vi "Test Asic Rate Scan Adders.vi"(8 "Error IN":errorcluster, 11 "Config Test IN":T2={"Config HW"={"VISA Rigol DP832"="Rigol_DP832", "Config Rigol DP832"=[{"Channel"=0, "V Limit"=5.5, "I Limit"=0.5, "V Out"=5.0}, {"Channel"=1, "V Limit"=5.5, "I Limit"=0.8, "V Out"=5.0}, {"Channel"=2, "V Limit"=5.5, "I Limit"=0.2, "V Out"=0.0}], "CTA Test#"="CTA013 A", "FT_Handle"=0, "Espera acceso FT"=10, "VISA Tek MDO3104"="Rigol_DP832", "VISA Key 81160A"="Rigol_DP832"}, "Config Test"=[{"Vasic"=2.8, "Global Reset"=FALSE, "Test Register?"=FALSE, "Test ADC?"=FALSE, "Test ADC"={"Repeats ADC"=100, "Max Desviation"=0.1}, "Limits ADC"={"Low"=[1.9, 1.3, 0.65, 0.0, 1.6, 1.4, 1.4, 0.9, 2.1, 0.85, 1.9], "High"=[2.1, 1.5, 0.85, 0.1, 1.4, 1.2, 1.2, 0.7, 1.9, 0.65, 1.7]}, "Test Max PN Min NP?"=FALSE, "Limits Max PN Min NP"={"Max P Upper"=2.177000045776367, "Min P Upper"=1.474, "Max N Upper"=1.475, "Min N Upper"=0.818, "Max P Lower"=1.888, "Min P Lower "=1.321, "Max N Lower"=1.322, "Min N Lower"=0.73}, "Test Rate Scan?"=FALSE, "Vin Rate Scan"=[], "Limits Rate Scan"={"High"=[0.15, 0.242, 0.331, 0.425, 0.512, 0.6, 0.688, 0.774, 0.847, 0.91], "Low"=[0.021, 0.11, 0.189, 0.27, 0.347, 0.421, 0.487, 0.551, 0.601, 0.635]}, "Test Rate Scan Adders?"=FALSE, "Vin Rate Adders"=[], "Limits Rate Scan adders"={"High"=[], "Low"=[]}, "Test offset analog?"=FALSE, "Lim Offset Analog"={"Max Analog"=0.05, "Min Analog"=-0.05}, "Test offset digital?"=FALSE, "Lim offset Dig"={"Max Dig"=0.05}, "Vasic real f.a."=2.8, "IBIAS"=FALSE, "VALUE IBIAS"=63}, {"Vasic"=2.8, "Global Reset"=FALSE, "Test Register?"=FALSE, "Test ADC?"=FALSE, "Test ADC"={"Repeats ADC"=100, "Max Desviation"=0.1}, "Limits ADC"={"Low"=[1.9, 1.3, 0.65, 0.0, 1.6, 1.4, 1.4, 0.9, 2.1, 0.85, 1.9], "High"=[2.1, 1.5, 0.85, 0.1, 1.4, 1.2, 1.2, 0.7, 1.9, 0.65, 1.7]}, "Test Max PN Min NP?"=FALSE, "Limits Max PN Min NP"={"Max P Upper"=2.177000045776367, "Min P Upper"=1.474, "Max N Upper"=1.475, "Min N Upper"=0.818, "Max P Lower"=1.888, "Min P Lower "=1.321, "Max N Lower"=1.322, "Min N Lower"=0.73}, "Test Rate Scan?"=FALSE, "Vin Rate Scan"=[], "Limits Rate Scan"={"High"=[0.15, 0.242, 0.331, 0.425, 0.512, 0.6, 0.688, 0.774, 0.847, 0.91], "Low"=[0.021, 0.11, 0.189, 0.27, 0.347, 0.421, 0.487, 0.551, 0.601, 0.635]}, "Test Rate Scan Adders?"=FALSE, "Vin Rate Adders"=[], "Limits Rate Scan adders"={"High"=[], "Low"=[]}, "Test offset analog?"=FALSE, "Lim Offset Analog"={"Max Analog"=0.05, "Min Analog"=-0.05}, "Test offset digital?"=FALSE, "Lim offset Dig"={"Max Dig"=0.05}, "Vasic real f.a."=2.8, "IBIAS"=FALSE, "VALUE IBIAS"=63}, {"Vasic"=2.8, "Global Reset"=FALSE, "Test Register?"=FALSE, "Test ADC?"=FALSE, "Test ADC"={"Repeats ADC"=100, "Max Desviation"=0.1}, "Limits ADC"={"Low"=[1.9, 1.3, 0.65, 0.0, 1.6, 1.4, 1.4, 0.9, 2.1, 0.85, 1.9], "High"=[2.1, 1.5, 0.85, 0.1, 1.4, 1.2, 1.2, 0.7, 1.9, 0.65, 1.7]}, "Test Max PN Min NP?"=FALSE, "Limits Max PN Min NP"={"Max P Upper"=2.177000045776367, "Min P Upper"=1.474, "Max N Upper"=1.475, "Min N Upper"=0.818, "Max P Lower"=1.888, "Min P Lower "=1.321, "Max N Lower"=1.322, "Min N Lower"=0.73}, "Test Rate Scan?"=FALSE, "Vin Rate Scan"=[], "Limits Rate Scan"={"High"=[0.15, 0.242, 0.331, 0.425, 0.512, 0.6, 0.688, 0.774, 0.847, 0.91], "Low"=[0.021, 0.11, 0.189, 0.27, 0.347, 0.421, 0.487, 0.551, 0.601, 0.635]}, "Test Rate Scan Adders?"=FALSE, "Vin Rate Adders"=[], "Limits Rate Scan adders"={"High"=[], "Low"=[]}, "Test offset analog?"=FALSE, "Lim Offset Analog"={"Max Analog"=0.05, "Min Analog"=-0.05}, "Test offset digital?"=FALSE, "Lim offset Dig"={"Max Dig"=0.05}, "Vasic real f.a."=2.8, "IBIAS"=FALSE, "VALUE IBIAS"=63}, {"Vasic"=2.8, "Global Reset"=FALSE, "Test Register?"=FALSE, "Test ADC?"=FALSE, "Test ADC"={"Repeats ADC"=100, "Max Desviation"=0.1}, "Limits ADC"={"Low"=[1.9, 1.3, 0.65, 0.0, 1.6, 1.4, 1.4, 0.9, 2.1, 0.85, 1.9], "High"=[2.1, 1.5, 0.85, 0.1, 1.4, 1.2, 1.2, 0.7, 1.9, 0.65, 1.7]}, "Test Max PN Min NP?"=FALSE, "Limits Max PN Min NP"={"Max P Upper"=2.177000045776367, "Min P Upper"=1.474, "Max N Upper"=1.475, "Min N Upper"=0.818, "Max P Lower"=1.888, "Min P Lower "=1.321, "Max N Lower"=1.322, "Min N Lower"=0.73}, "Test Rate Scan?"=FALSE, "Vin Rate Scan"=[], "Limits Rate Scan"={"High"=[0.15, 0.242, 0.331, 0.425, 0.512, 0.6, 0.688, 0.774, 0.847, 0.91], "Low"=[0.021, 0.11, 0.189, 0.27, 0.347, 0.421, 0.487, 0.551, 0.601, 0.635]}, "Test Rate Scan Adders?"=FALSE, "Vin Rate Adders"=[], "Limits Rate Scan adders"={"High"=[], "Low"=[]}, "Test offset analog?"=FALSE, "Lim Offset Analog"={"Max Analog"=0.05, "Min Analog"=-0.05}, "Test offset digital?"=FALSE, "Lim offset Dig"={"Max Dig"=0.05}, "Vasic real f.a."=2.8, "IBIAS"=FALSE, "VALUE IBIAS"=63}], "Result"=[], "Execucion Test"={"Vasic Actual"=0}, "Config VGA"={"Theoretical Voltage"=[], "Real Voltage"=[102.85, 207.14, 299.57, 404.85, 495.71, 606.85, 697.71, 801.14, 897.14, 998.85], "Pulse Width"=57344, "Frecuency Pulse"=1000000.0, "VGA Gain"=[9, 16, 24, 34, 43, 52, 61, 72, 81, 93]}, "Test Info"={"Asic"="", "Operator"="", "Place"="", "Time start"=timestamp(0 s since 1904-01-01), "Time stop"=timestamp(0 s since 1904-01-01)}, "Info machine"={"SO"="", "SO Name"="", "SO Ver"="", "SO Build"="", "CPU"="", "APP"="", "APP YEAR"="", "APP ver"="", "APP User"="", "APP Serail"="", "MAC"=[], "PC NAME"=[], "PC IP"=[], "BIOS MANU"="", "BIOS NAME"="", "BIOS SERIAL"="", "BOARD MANU"="", "BOARD NAME"="", "BOARD SERIAL"="", "Driver Version"="", "Library Version"="", "FPGA Ver"=0, "ID CTA board"=0, "LAST BOOT"="", "LABVIEW Ver"=0}, "Partial Report"="", "CONFIG GEN"=[]} {"CONFIG GEN"."Vasic Theorical" min=1.0 max=1000000.0 step=1.0 format="%#_6pV"; "CONFIG GEN"."Frequency" min=0.001 max=333000000.0 step=1000.0 format="%#_6pHz"; "CONFIG GEN"."Leading Edge Time" min=1e-09 max=1.0 step=1e-10 format="%#_6ps"; "CONFIG GEN"."Trailing Edge Time" min=1e-09 max=1.0 step=1e-10 format="%#_6ps"; "CONFIG GEN"."Delay" min=0.0 max=1.0 step=1e-12 format="%#_6ps"; "CONFIG GEN"."Trigger Level Sync" items=["ECL", "TTL"]; "CONFIG GEN"."Trigger Sync Out" items=["AB"=3, "B"=2, "A"=1, "None"=0]; "CONFIG GEN"."Load" min=1.0 max=1000000.0 step=1.0 format="%#_6p"; "CONFIG GEN"."DC Offset" min=-10.0 max=10.0 step=0.1 format="%#_6pV"; "CONFIG GEN"."Amplitude" min=0.05 max=5.0 step=0.001 format="%#_6pV"; "CONFIG GEN"."Width Time" min=1.5e-09 max=1.0 step=1e-10 format="%#_6ps"; "CONFIG GEN"."Channel" items=["Channel1"=1, "Channel2"=2]; "Config VGA"."Theoretical Voltage" format="%1.4f"; "Config VGA"."VGA Gain" format="%02x"; "Config VGA"."Frecuency Pulse" format="%0_2p"; "Config VGA"."Pulse Width" format="%04x"; "Config VGA"."Real Voltage" format="%1.5f"; "Config Test"."VALUE IBIAS" max=63 step=1; "Config Test"."Vasic real f.a." min=2.8 max=3.8 step=0.01 format="%.2g"; "Config Test"."Limits Rate Scan adders"."Low" format="%1.3f"; "Config Test"."Limits Rate Scan adders"."High" format="%1.3f"; "Config Test"."Limits ADC"."High" format="%1.4f"; "Config Test"."Limits ADC"."Low" format="%1.3f"; "Config Test"."Lim offset Dig"."Max Dig" format="%.3g"; "Config Test"."Lim Offset Analog"."Min Analog" format="%.3g"; "Config Test"."Lim Offset Analog"."Max Analog" format="%.3g"; "Config Test"."Limits Rate Scan"."Low" format="%1.4f"; "Config Test"."Limits Rate Scan"."High" format="%1.3f"; "Config Test"."Limits Max PN Min NP"."Min P Upper" format="%.3g"; "Config Test"."Limits Max PN Min NP"."Min P Lower" format="%.3g"; "Config Test"."Limits Max PN Min NP"."Max N Lower" format="%.3g"; "Config Test"."Limits Max PN Min NP"."Max N Upper" format="%.3g"; "Config Test"."Limits Max PN Min NP"."Min N Lower" format="%.3g"; "Config Test"."Limits Max PN Min NP"."Min N Upper" format="%.3g"; "Config Test"."Limits Max PN Min NP"."Max P Upper" format="%.3g"; "Config Test"."Limits Max PN Min NP"."Max P Lower" format="%.3g"; "Config Test"."Vasic" min=2.8 max=3.8 step=0.01 format="%.2g"; "Config HW"."Config Rigol DP832"."Channel" items=["+30V Channel 1", "+30V Channel 2", "+5V Channel 3"]; "Config HW"."Config Rigol DP832"."V Limit" format="%.1g"; "Config HW"."Config Rigol DP832"."I Limit" format="%.1g"; "Config HW"."Config Rigol DP832"."V Out" format="%.1g"; "Result"."Test Registros"."Read W/R" format="%04x"; "Result"."Test Registros"."Pattern W/R" format="%04x"; "Result"."Test Registros"."Read Default" format="%04x"; "Result"."Test Registros"."Pattern Default" format="%04x"}) -> (0 "Error OUT":errorcluster, 2 "Rate scan adders all ok":bool, 3 "Config Test OUT":T2={"Config HW"={"VISA Rigol DP832"="Rigol_DP832", "Config Rigol DP832"=[{"Channel"=0, "V Limit"=5.5, "I Limit"=0.5, "V Out"=5.0}, {"Channel"=1, "V Limit"=5.5, "I Limit"=0.8, "V Out"=5.0}, {"Channel"=2, "V Limit"=5.5, "I Limit"=0.2, "V Out"=0.0}], "CTA Test#"="CTA013 A", "FT_Handle"=0, "Espera acceso FT"=10, "VISA Tek MDO3104"="Rigol_DP832", "VISA Key 81160A"="Rigol_DP832"}, "Config Test"=[{"Vasic"=2.8, "Global Reset"=FALSE, "Test Register?"=FALSE, "Test ADC?"=FALSE, "Test ADC"={"Repeats ADC"=100, "Max Desviation"=0.1}, "Limits ADC"={"Low"=[1.9, 1.3, 0.65, 0.0, 1.6, 1.4, 1.4, 0.9, 2.1, 0.85, 1.9], "High"=[2.1, 1.5, 0.85, 0.1, 1.4, 1.2, 1.2, 0.7, 1.9, 0.65, 1.7]}, "Test Max PN Min NP?"=FALSE, "Limits Max PN Min NP"={"Max P Upper"=2.177000045776367, "Min P Upper"=1.474, "Max N Upper"=1.475, "Min N Upper"=0.818, "Max P Lower"=1.888, "Min P Lower "=1.321, "Max N Lower"=1.322, "Min N Lower"=0.73}, "Test Rate Scan?"=FALSE, "Vin Rate Scan"=[], "Limits Rate Scan"={"High"=[0.15, 0.242, 0.331, 0.425, 0.512, 0.6, 0.688, 0.774, 0.847, 0.91], "Low"=[0.021, 0.11, 0.189, 0.27, 0.347, 0.421, 0.487, 0.551, 0.601, 0.635]}, "Test Rate Scan Adders?"=FALSE, "Vin Rate Adders"=[], "Limits Rate Scan adders"={"High"=[], "Low"=[]}, "Test offset analog?"=FALSE, "Lim Offset Analog"={"Max Analog"=0.05, "Min Analog"=-0.05}, "Test offset digital?"=FALSE, "Lim offset Dig"={"Max Dig"=0.05}, "Vasic real f.a."=2.8, "IBIAS"=FALSE, "VALUE IBIAS"=63}, {"Vasic"=2.8, "Global Reset"=FALSE, "Test Register?"=FALSE, "Test ADC?"=FALSE, "Test ADC"={"Repeats ADC"=100, "Max Desviation"=0.1}, "Limits ADC"={"Low"=[1.9, 1.3, 0.65, 0.0, 1.6, 1.4, 1.4, 0.9, 2.1, 0.85, 1.9], "High"=[2.1, 1.5, 0.85, 0.1, 1.4, 1.2, 1.2, 0.7, 1.9, 0.65, 1.7]}, "Test Max PN Min NP?"=FALSE, "Limits Max PN Min NP"={"Max P Upper"=2.177000045776367, "Min P Upper"=1.474, "Max N Upper"=1.475, "Min N Upper"=0.818, "Max P Lower"=1.888, "Min P Lower "=1.321, "Max N Lower"=1.322, "Min N Lower"=0.73}, "Test Rate Scan?"=FALSE, "Vin Rate Scan"=[], "Limits Rate Scan"={"High"=[0.15, 0.242, 0.331, 0.425, 0.512, 0.6, 0.688, 0.774, 0.847, 0.91], "Low"=[0.021, 0.11, 0.189, 0.27, 0.347, 0.421, 0.487, 0.551, 0.601, 0.635]}, "Test Rate Scan Adders?"=FALSE, "Vin Rate Adders"=[], "Limits Rate Scan adders"={"High"=[], "Low"=[]}, "Test offset analog?"=FALSE, "Lim Offset Analog"={"Max Analog"=0.05, "Min Analog"=-0.05}, "Test offset digital?"=FALSE, "Lim offset Dig"={"Max Dig"=0.05}, "Vasic real f.a."=2.8, "IBIAS"=FALSE, "VALUE IBIAS"=63}, {"Vasic"=2.8, "Global Reset"=FALSE, "Test Register?"=FALSE, "Test ADC?"=FALSE, "Test ADC"={"Repeats ADC"=100, "Max Desviation"=0.1}, "Limits ADC"={"Low"=[1.9, 1.3, 0.65, 0.0, 1.6, 1.4, 1.4, 0.9, 2.1, 0.85, 1.9], "High"=[2.1, 1.5, 0.85, 0.1, 1.4, 1.2, 1.2, 0.7, 1.9, 0.65, 1.7]}, "Test Max PN Min NP?"=FALSE, "Limits Max PN Min NP"={"Max P Upper"=2.177000045776367, "Min P Upper"=1.474, "Max N Upper"=1.475, "Min N Upper"=0.818, "Max P Lower"=1.888, "Min P Lower "=1.321, "Max N Lower"=1.322, "Min N Lower"=0.73}, "Test Rate Scan?"=FALSE, "Vin Rate Scan"=[], "Limits Rate Scan"={"High"=[0.15, 0.242, 0.331, 0.425, 0.512, 0.6, 0.688, 0.774, 0.847, 0.91], "Low"=[0.021, 0.11, 0.189, 0.27, 0.347, 0.421, 0.487, 0.551, 0.601, 0.635]}, "Test Rate Scan Adders?"=FALSE, "Vin Rate Adders"=[], "Limits Rate Scan adders"={"High"=[], "Low"=[]}, "Test offset analog?"=FALSE, "Lim Offset Analog"={"Max Analog"=0.05, "Min Analog"=-0.05}, "Test offset digital?"=FALSE, "Lim offset Dig"={"Max Dig"=0.05}, "Vasic real f.a."=2.8, "IBIAS"=FALSE, "VALUE IBIAS"=63}, {"Vasic"=2.8, "Global Reset"=FALSE, "Test Register?"=FALSE, "Test ADC?"=FALSE, "Test ADC"={"Repeats ADC"=100, "Max Desviation"=0.1}, "Limits ADC"={"Low"=[1.9, 1.3, 0.65, 0.0, 1.6, 1.4, 1.4, 0.9, 2.1, 0.85, 1.9], "High"=[2.1, 1.5, 0.85, 0.1, 1.4, 1.2, 1.2, 0.7, 1.9, 0.65, 1.7]}, "Test Max PN Min NP?"=FALSE, "Limits Max PN Min NP"={"Max P Upper"=2.177000045776367, "Min P Upper"=1.474, "Max N Upper"=1.475, "Min N Upper"=0.818, "Max P Lower"=1.888, "Min P Lower "=1.321, "Max N Lower"=1.322, "Min N Lower"=0.73}, "Test Rate Scan?"=FALSE, "Vin Rate Scan"=[], "Limits Rate Scan"={"High"=[0.15, 0.242, 0.331, 0.425, 0.512, 0.6, 0.688, 0.774, 0.847, 0.91], "Low"=[0.021, 0.11, 0.189, 0.27, 0.347, 0.421, 0.487, 0.551, 0.601, 0.635]}, "Test Rate Scan Adders?"=FALSE, "Vin Rate Adders"=[], "Limits Rate Scan adders"={"High"=[], "Low"=[]}, "Test offset analog?"=FALSE, "Lim Offset Analog"={"Max Analog"=0.05, "Min Analog"=-0.05}, "Test offset digital?"=FALSE, "Lim offset Dig"={"Max Dig"=0.05}, "Vasic real f.a."=2.8, "IBIAS"=FALSE, "VALUE IBIAS"=63}], "Result"=[], "Execucion Test"={"Vasic Actual"=0}, "Config VGA"={"Theoretical Voltage"=[], "Real Voltage"=[102.85, 207.14, 299.57, 404.85, 495.71, 606.85, 697.71, 801.14, 897.14, 998.85], "Pulse Width"=57344, "Frecuency Pulse"=1000000.0, "VGA Gain"=[9, 16, 24, 34, 43, 52, 61, 72, 81, 93]}, "Test Info"={"Asic"="", "Operator"="", "Place"="", "Time start"=timestamp(0 s since 1904-01-01), "Time stop"=timestamp(0 s since 1904-01-01)}, "Info machine"={"SO"="", "SO Name"="", "SO Ver"="", "SO Build"="", "CPU"="", "APP"="", "APP YEAR"="", "APP ver"="", "APP User"="", "APP Serail"="", "MAC"=[], "PC NAME"=[], "PC IP"=[], "BIOS MANU"="", "BIOS NAME"="", "BIOS SERIAL"="", "BOARD MANU"="", "BOARD NAME"="", "BOARD SERIAL"="", "Driver Version"="", "Library Version"="", "FPGA Ver"=0, "ID CTA board"=0, "LAST BOOT"="", "LABVIEW Ver"=0}, "Partial Report"="", "CONFIG GEN"=[]} {"CONFIG GEN"."Vasic Theorical" min=1.0 max=1000000.0 step=1.0 format="%#_6pV"; "CONFIG GEN"."Frequency" min=0.001 max=333000000.0 step=1000.0 format="%#_6pHz"; "CONFIG GEN"."Leading Edge Time" min=1e-09 max=1.0 step=1e-10 format="%#_6ps"; "CONFIG GEN"."Trailing Edge Time" min=1e-09 max=1.0 step=1e-10 format="%#_6ps"; "CONFIG GEN"."Delay" min=0.0 max=1.0 step=1e-12 format="%#_6ps"; "CONFIG GEN"."Trigger Level Sync" items=["ECL", "TTL"]; "CONFIG GEN"."Trigger Sync Out" items=["AB"=3, "B"=2, "A"=1, "None"=0]; "CONFIG GEN"."Load" min=1.0 max=1000000.0 step=1.0 format="%#_6p"; "CONFIG GEN"."DC Offset" min=-10.0 max=10.0 step=0.1 format="%#_6pV"; "CONFIG GEN"."Amplitude" min=0.05 max=5.0 step=0.001 format="%#_6pV"; "CONFIG GEN"."Width Time" min=1.5e-09 max=1.0 step=1e-10 format="%#_6ps"; "CONFIG GEN"."Channel" items=["Channel1"=1, "Channel2"=2]; "Config VGA"."Theoretical Voltage" format="%1.4f"; "Config VGA"."VGA Gain" format="%02x"; "Config VGA"."Frecuency Pulse" format="%0_2p"; "Config VGA"."Pulse Width" format="%04x"; "Config VGA"."Real Voltage" format="%1.5f"; "Config Test"."VALUE IBIAS" max=63 step=1; "Config Test"."Vasic real f.a." min=2.8 max=3.8 step=0.01 format="%.2g"; "Config Test"."Limits Rate Scan adders"."Low" format="%1.3f"; "Config Test"."Limits Rate Scan adders"."High" format="%1.3f"; "Config Test"."Limits ADC"."High" format="%1.4f"; "Config Test"."Limits ADC"."Low" format="%1.3f"; "Config Test"."Lim offset Dig"."Max Dig" format="%.3g"; "Config Test"."Lim Offset Analog"."Min Analog" format="%.3g"; "Config Test"."Lim Offset Analog"."Max Analog" format="%.3g"; "Config Test"."Limits Rate Scan"."Low" format="%1.4f"; "Config Test"."Limits Rate Scan"."High" format="%1.3f"; "Config Test"."Limits Max PN Min NP"."Min P Upper" format="%.3g"; "Config Test"."Limits Max PN Min NP"."Min P Lower" format="%.3g"; "Config Test"."Limits Max PN Min NP"."Max N Lower" format="%.3g"; "Config Test"."Limits Max PN Min NP"."Max N Upper" format="%.3g"; "Config Test"."Limits Max PN Min NP"."Min N Lower" format="%.3g"; "Config Test"."Limits Max PN Min NP"."Min N Upper" format="%.3g"; "Config Test"."Limits Max PN Min NP"."Max P Upper" format="%.3g"; "Config Test"."Limits Max PN Min NP"."Max P Lower" format="%.3g"; "Config Test"."Vasic" min=2.8 max=3.8 step=0.01 format="%.2g"; "Config HW"."Config Rigol DP832"."Channel" items=["+30V Channel 1", "+30V Channel 2", "+5V Channel 3"]; "Config HW"."Config Rigol DP832"."V Limit" format="%.1g"; "Config HW"."Config Rigol DP832"."I Limit" format="%.1g"; "Config HW"."Config Rigol DP832"."V Out" format="%.1g"; "Result"."Test Registros"."Read W/R" format="%04x"; "Result"."Test Registros"."Pattern W/R" format="%04x"; "Result"."Test Registros"."Read Default" format="%04x"; "Result"."Test Registros"."Pattern Default" format="%04x"})   [LabVIEW 2019]
uses:
  Test.ctl
  TEST.TEST CONFIG HW.ctl
  Rigol DP832/DP832_Control Channels.ctl
  TEST.TEST CONFIG TEST MATRIZ.ctl
  TEST.TEST CONFIG TEST.ctl
  TEST.TEST RESULT.ctl
  test_result fvasic.ctl
  TEST.TEST EXECUTION TEST.ctl
  TEST.TEST CONFIG VGA.ctl
  TEST.TEST TEST INFO.ctl
  TEST.TEST INFO PC.ctl
  GenPulse_configurar.ctl
  Global.Salir Ya.vi
panel:
  out "Vin real gen":dbl[](array[numeric])
  in  "Debug":enum32{"Page 1", "Page 2"}(tab)
  in  "Operacion":enum32{"Page 1", "Page 2"}(tab)
  out "%":u8 format="%02d%%"
  out "B":u8(slide) scale=0.0..100.0
  out "Indicador":string
  out "HLTHx":dbl
  out "LLTHx":dbl
  out "WRITE OK":bool
  out "Amplitude":dbl
  in  "Column Headers":string[](array[string])=["MODE 2 (2+4)", "MODE 2 (3+4)", "MODE 2 (4+5)", "MODE 3 (2+3+4)", "MODE 3 (3+4+5)", "MODE 3 (4+5+6)", "MODE 4 (2+3+4+5)", "MODE 4 (3+4+5+6)", "MODE 4 (1+4+5+6)"]
  out "DAC TH0,TH1,TH2 2":u16[][][](array[numeric])
  out "DAC TH3,TH4,TH5 2":u16[][][](array[numeric])
  out "Volt HLTH":dbl[][][](array[numeric])
  out "Volt LLTH":dbl[][][](array[numeric])
  out "DAC TH0,TH1,TH2":u16
  out "DAC TH3,TH4,TH5":u16
  out "Comparation HLTH":bool[][][](array[boolean])
  out "Comparation LLTH":bool[][][](array[boolean])
  out "Ref":T1
  out "Salida A rectificada":dbl[][][](array[numeric])
  out "Cruze por 0 Salida A":dbl[][](array[numeric])
  out "Cruze por 0 Salida B":dbl[][](array[numeric])
  out "Salida B rectificada":dbl[][][](array[numeric])
  out "HIGH":dbl[][](array[numeric])
  out "LOW":dbl[][](array[numeric])
  out "Vasic theo":dbl[](array[numeric])
  out "logical AND":bool
  out "logical AND 2":bool
  out "Volt HLTH Corregido":dbl[](array[numeric])
  out "Volt LLTH Corregido":dbl[](array[numeric])
  out "low":dbl
  out "h8ig":dbl
  # "Vin Asic\nMode"
  # "Vin Asic\nMode"
  # "VIN\nMODE\nCHANELL"
  # "???"
  # "???"
  # "???"
  # "VIN\nMODE\nCHANELL"
  # "???"
  # "Test ASIC. Rate Scan Adders"
  # "Modo 2\nModo 3\nModo 4\nModo 2\nModo 3\nModo 4"
  # "Modo 2\nModo 3\nModo 4\nModo 2\nModo 3\nModo 4"
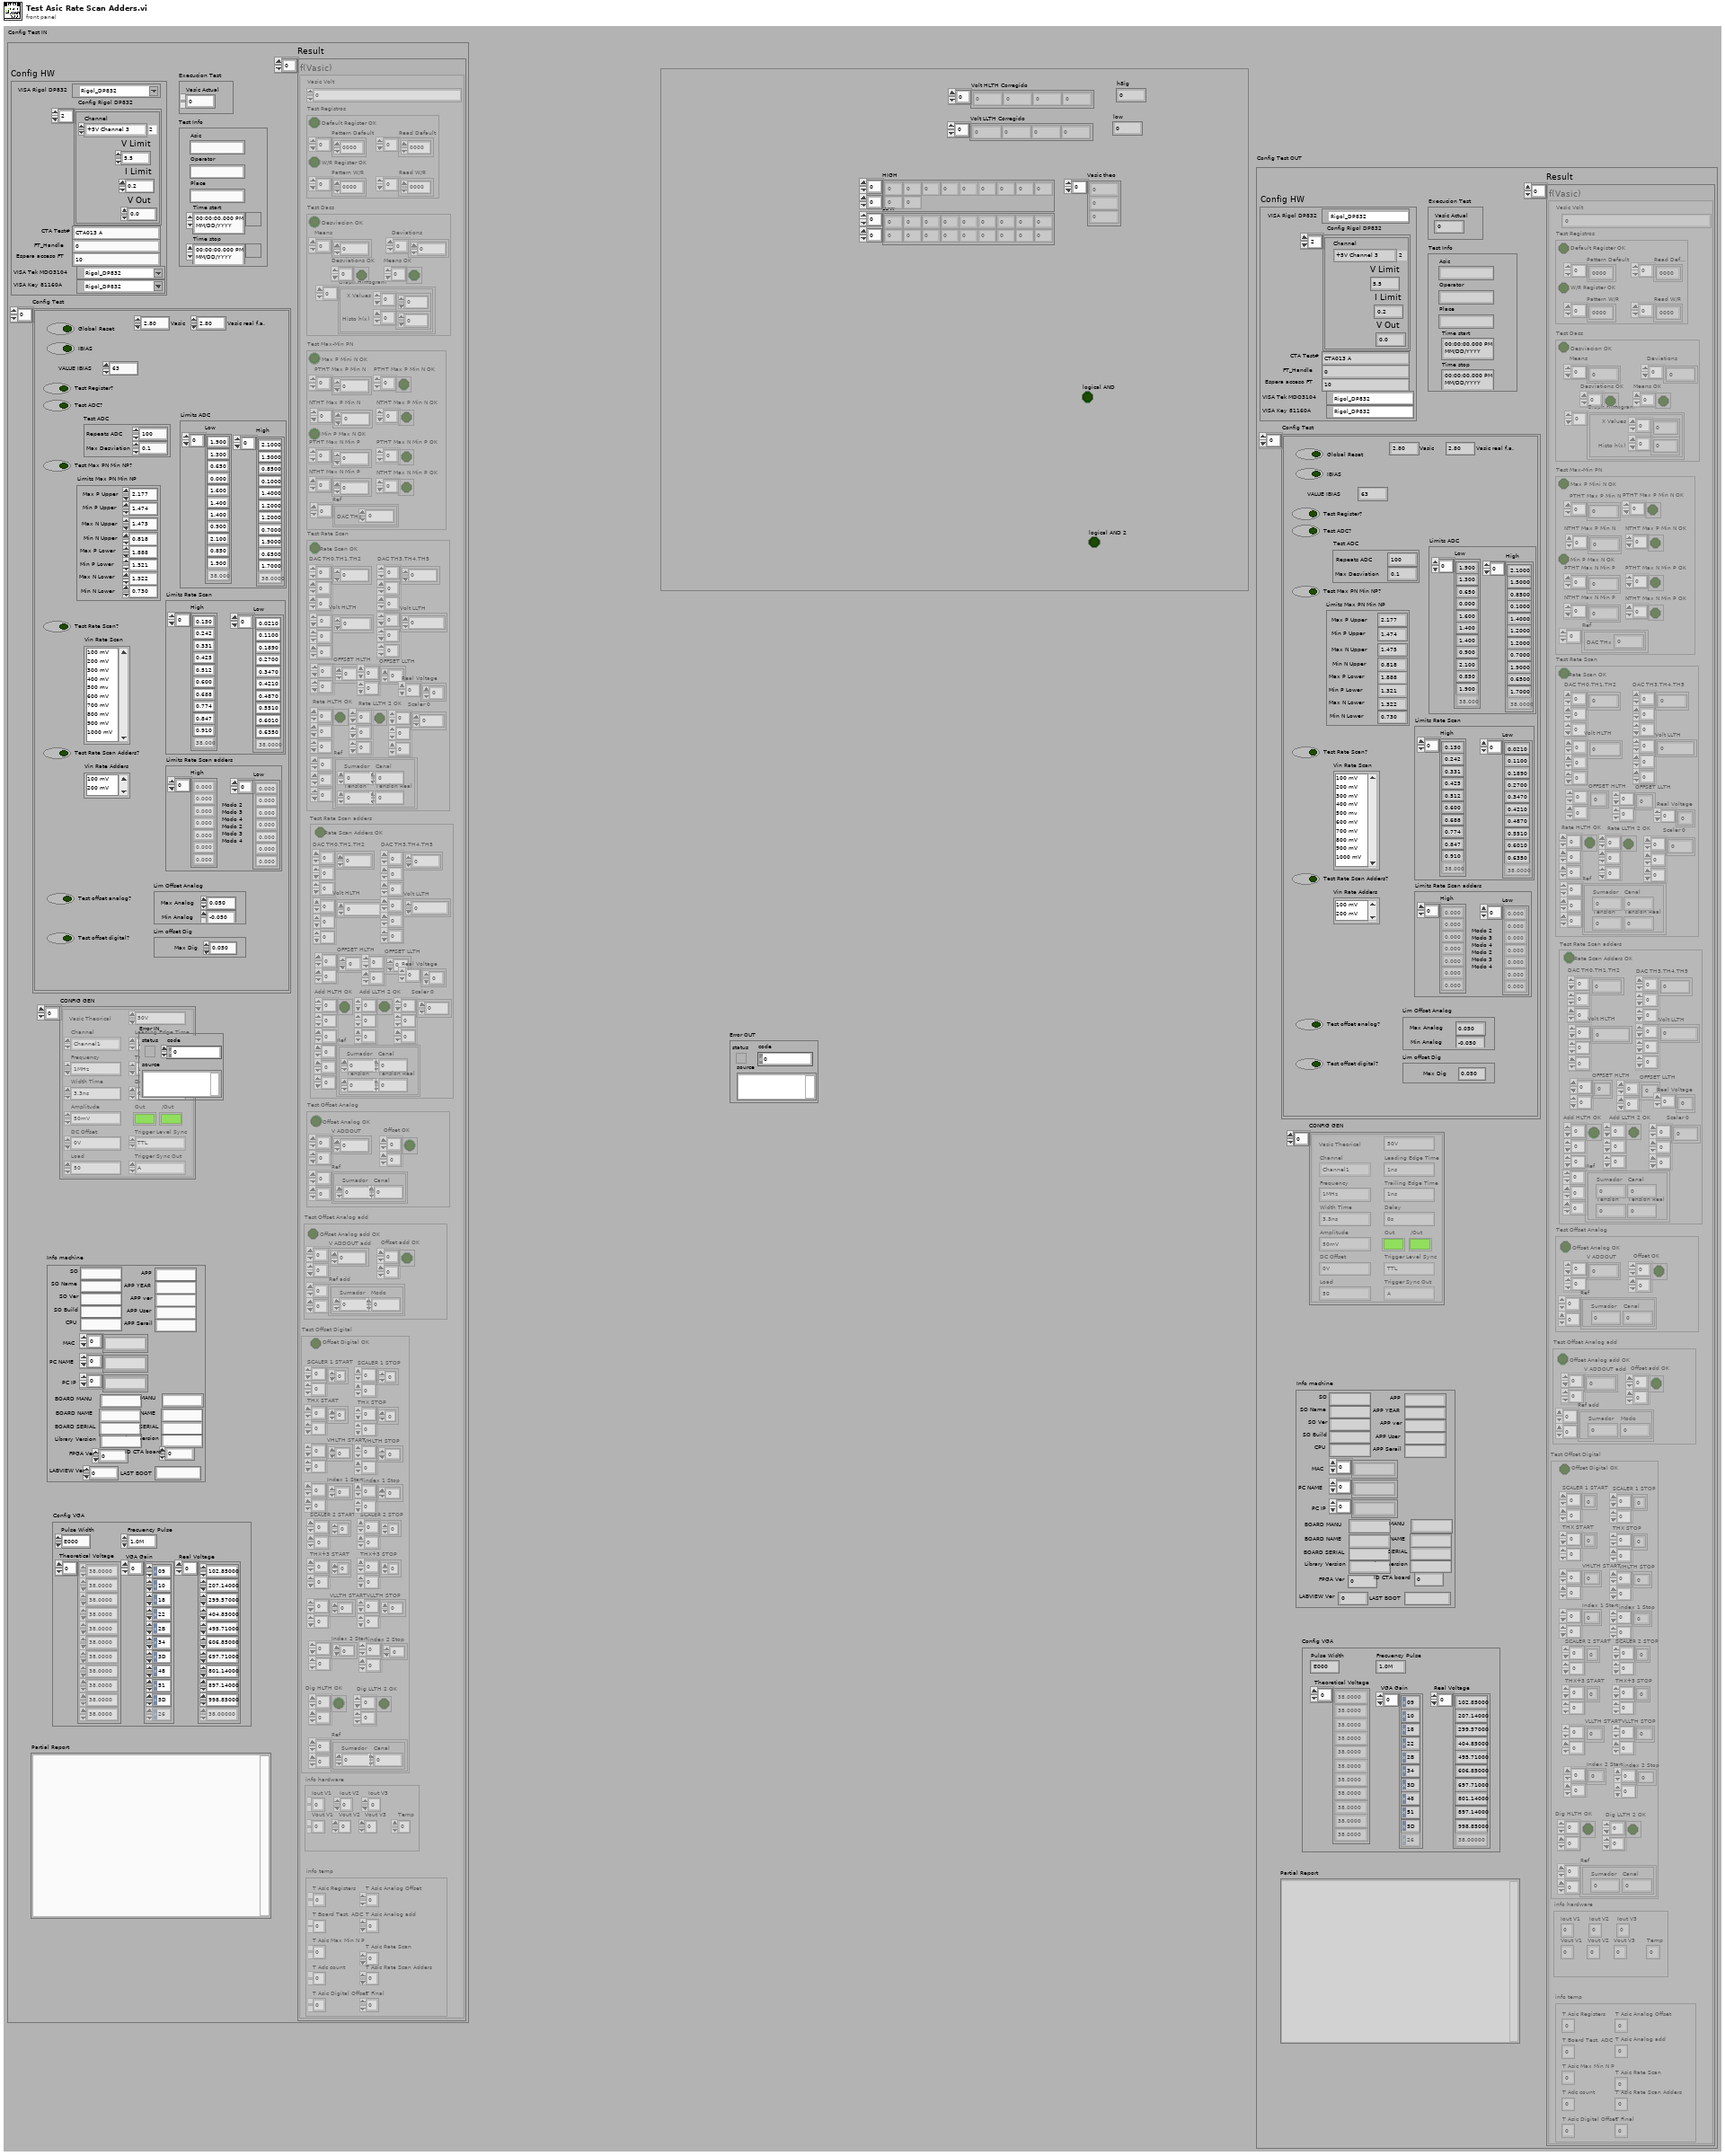
[diagram p1: front panel]
types:
  T1 = cluster{"Sumador":u8, "Modo":u8, "Tension":u8, "Tension Real":dbl}
  T2 = typedef "Test.ctl" = cluster{"Config HW":T3, "Config Test":T5, "Result":T7, "Execucion Test":T9, "Config VGA":T10, "Test Info":T11, "Info machine":T12, "Partial Report":string, "CONFIG GEN":T13[]}
  T3 = typedef "TEST.TEST CONFIG HW.ctl" = cluster{"VISA Rigol DP832":refnum<visa-resource-name>, "Config Rigol DP832":cluster{"Channel":T4, "V Limit":dbl, "I Limit":dbl, "V Out":dbl}[], "CTA Test#":string, "FT_Handle":u32, "Espera acceso FT":u32, "VISA Tek MDO3104":refnum<visa-resource-name>, "VISA Key 81160A":refnum<visa-resource-name>}
  T4 = typedef "DP832_Control Channels.ctl" = i32
  T5 = typedef "TEST.TEST CONFIG TEST MATRIZ.ctl" = T6[]
  T6 = typedef "TEST.TEST CONFIG TEST.ctl" = cluster{"Vasic":dbl, "Global Reset":bool, "Test Register?":bool, "Test ADC?":bool, "Test ADC":cluster{"Repeats ADC":i32, "Max Desviation":dbl}, "Limits ADC":cluster{"Low":dbl[], "High":dbl[]}, "Test Max PN Min NP?":bool, "Limits Max PN Min NP":cluster{"Max P Upper":dbl, "Min P Upper":dbl, "Max N Upper":dbl, "Min N Upper":dbl, "Max P Lower":dbl, "Min P Lower ":dbl, "Max N Lower":dbl, "Min N Lower":dbl}, "Test Rate Scan?":bool, "Vin Rate Scan":i32[], "Limits Rate Scan":cluster{"High":dbl[], "Low":dbl[]}, "Test Rate Scan Adders?":bool, "Vin Rate Adders":i32[], "Limits Rate Scan adders":cluster{"High":dbl[], "Low":dbl[]}, "Test offset analog?":bool, "Lim Offset Analog":cluster{"Max Analog":dbl, "Min Analog":dbl}, "Test offset digital?":bool, "Lim offset Dig":cluster{"Max Dig":dbl}, "Vasic real f.a.":dbl, "IBIAS":bool, "VALUE IBIAS":u8}
  T7 = typedef "TEST.TEST RESULT.ctl" = T8[]
  T8 = typedef "test_result fvasic.ctl" = cluster{"Vasic Volt":i32, "Test Registros":cluster{"Default Register OK":bool, "Pattern Default":u16[], "Read Default":u16[], "W/R Register OK":bool, "Pattern W/R":u16[], "Read W/R":u16[]}, "Test Dacs":cluster{"Desviacion OK":bool, "Means":dbl[], "Deviations":dbl[], "Desviations OK":bool[], "Means OK":bool[], "Graph Histogram":cluster{"X Values":dbl[], "Histo h(x)":i32[]}[]}, "Test Max-Min PN":cluster{"Max P Mini N OK":bool, "PTHT Max P Min N":dbl[], "PTHT Max P Min N OK":bool[], "NTHT Max P Min N":dbl[], "NTHT Max P Min N OK":bool[], "Min P Max N OK":bool, "PTHT Max N Min P":dbl[], "PTHT Max N Min P OK":bool[], "NTHT Max N Min P":dbl[], "NTHT Max N Min P OK":bool[], "Ref":cluster{"DAC THx":u8}[]}, "Test Rate Scan":cluster{"Rate Scan OK":bool, "DAC TH0,TH1,TH2":u16[][][], "Volt HLTH":dbl[][][], "Rate HLTH OK":bool[][][], "DAC TH3,TH4,TH5":u16[][][], "Volt LLTH":dbl[][][], "Rate LLTH 2 OK":bool[][][], "Scaler 0":u16[][][], "Ref":cluster{"Sumador":u8, "Canal":u8, "Tension":u8, "Tension Real":dbl}[][][], "OFFSET HLTH":dbl[][], "OFFSET LLTH":dbl[][], "Real Voltage":dbl[]}, "Test Rate Scan adders":cluster{"Rate Scan Adders OK":bool, "DAC TH0,TH1,TH2":u16[][][], "Volt HLTH":dbl[][][], "Add HLTH OK":bool[][][], "DAC TH3,TH4,TH5":u16[][][], "Volt LLTH":dbl[][][], "Add LLTH 2 OK":bool[][][], "Scaler 0":u16[][][], "Ref":cluster{"Sumador":u8, "Canal":u8, "Tension":u8, "Tension Real":dbl}[][][], "OFFSET HLTH":dbl[][], "OFFSET LLTH":dbl[][], "Real Voltage":dbl[]}, "Test Offset Analog":cluster{"Offset Analog OK":bool, "V ADDOUT":dbl[][], "Offset OK":bool[][], "Ref":cluster{"Sumador":u8, "Canal":u8}[][]}, "Test Offset Digital":cluster{"Offset Digital OK":bool, "SCALER 1 START":u16[][], "SCALER 1 STOP":u16[][], "THX START":u16[][], "THX STOP":u16[][], "VHLTH START":dbl[][], "VHLTH STOP":dbl[][], "Index 1 Start":i32[][], "index 1 Stop":i32[][], "SCALER 2 START":u16[][], "SCALER 2 STOP":u16[][], "THX+3 START":u16[][], "THX+3 STOP":u16[][], "VLLTH START":dbl[][], "VLLTH STOP":dbl[][], "Index 2 Start":i32[][], "index 2 Stop":i32[][], "Dig HLTH OK":bool[][], "Dig LLTH 2 OK":bool[][], "Ref":cluster{"Sumador":u8, "Canal":u8}[][]}, "info hardware":cluster{"Iout V1":dbl, "Iout V2":dbl, "Iout V3":dbl, "Vout V1":dbl, "Vout V2":dbl, "Vout V3":dbl, "Temp":dbl}, "Test Offset Analog add":cluster{"Offset Analog add OK":bool, "V ADDOUT add":dbl[][], "Offset add OK":bool[][], "Ref add":cluster{"Sumador":u8, "Modo":u8}[][]}, "info temp":cluster{"T Asic Registers":dbl, "T Board Test. ADC":dbl, "T Asic Max Min N P":dbl, "T Adc count":dbl, "T Asic Digital Offset":dbl, "T Asic Analog Offset":dbl, "T Asic Analog add":dbl, "T Asic Rate Scan":dbl, "T Asic Rate Scan Adders":dbl, "T Final":dbl}}
  T9 = typedef "TEST.TEST EXECUTION TEST.ctl" = cluster{"Vasic Actual":i32}
  T10 = typedef "TEST.TEST CONFIG VGA.ctl" = cluster{"Theoretical Voltage":dbl[], "Real Voltage":dbl[], "Pulse Width":u16, "Frecuency Pulse":dbl, "VGA Gain":u8[]}
  T11 = typedef "TEST.TEST TEST INFO.ctl" = cluster{"Asic":string, "Operator":string, "Place":string, "Time start":timestamp, "Time stop":timestamp}
  T12 = typedef "TEST.TEST INFO PC.ctl" = cluster{"SO":string, "SO Name":string, "SO Ver":string, "SO Build":string, "CPU":string, "APP":string, "APP YEAR":string, "APP ver":string, "APP User":string, "APP Serail":string, "MAC":string[], "PC NAME":string[], "PC IP":string[], "BIOS MANU":string, "BIOS NAME":string, "BIOS SERIAL":string, "BOARD MANU":string, "BOARD NAME":string, "BOARD SERIAL":string, "Driver Version":string, "Library Version":string, "FPGA Ver":u8, "ID CTA board":u64, "LAST BOOT":string, "LABVIEW Ver":u32}
  T13 = typedef "GenPulse_configurar.ctl" = cluster{"Channel":u16, "Frequency":dbl, "Width Time":dbl, "Amplitude":dbl, "DC Offset":dbl, "Load":dbl, "Leading Edge Time":dbl, "Trailing Edge Time":dbl, "Delay":dbl, "Out":bool, "/Out":bool, "Trigger Level Sync":u16, "Trigger Sync Out":u16, "Vasic Theorical":dbl}
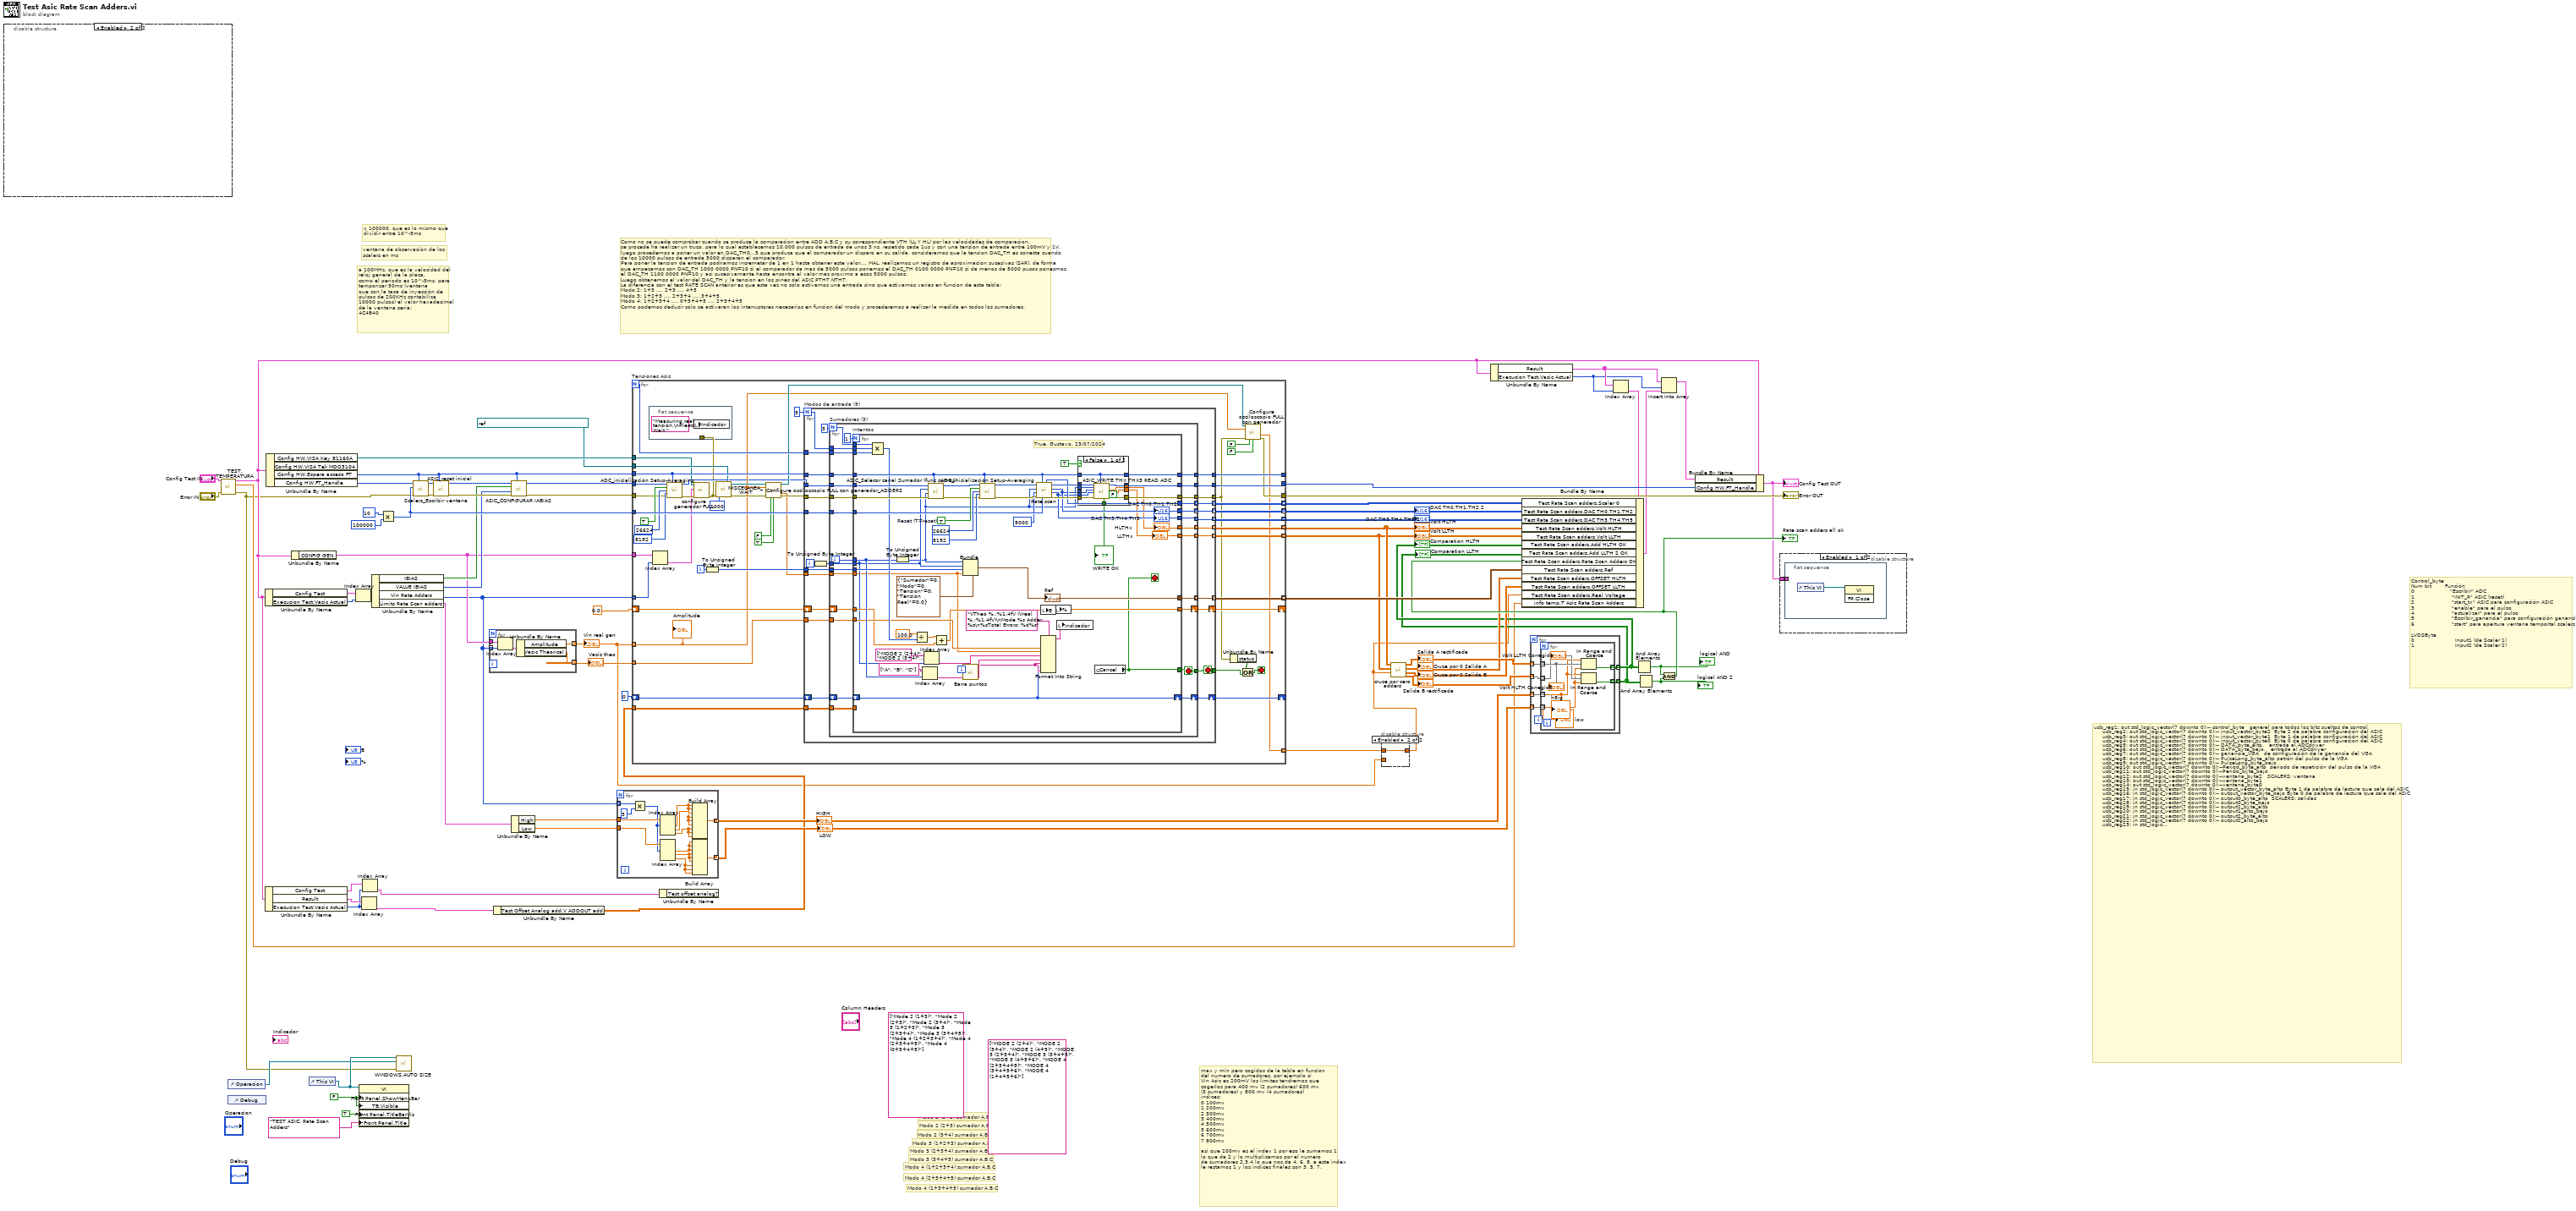
[diagram p0: block diagram]
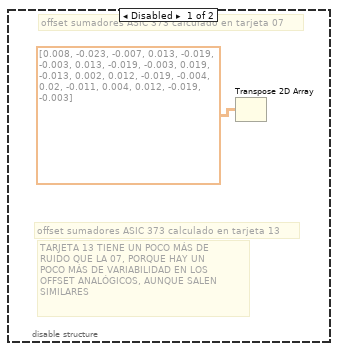
[diagram p4: hidden frame]
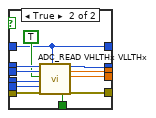
[diagram p5: hidden frame]
diagram:
  (unwired) string[] ["MODE 2 (2+4)", "MODE 2 (3+4)", "MODE 2 (4+5)", "MODE 3 (2+3+4)", "MODE 3 (3+4+5)", "MODE 3 (4+5+6)", "MODE 4 (2+3+4+5)", "MODE 4 (3+4+5+6)", "MODE 4 (1+4+5+6)"] ("Column Headers")
  (unwired) string[] ["Mode 2 (1+3)", "Mode 2 (2+3)", "Mode 2 (3+4)", "Mode 3 (1+2+3)", "Mode 3 (2+3+4)", "Mode 3 (3+4+5)", "Mode 4 (1+2+3+4)", "Mode 4 (2+3+4+5)", "Mode 4 (0+3+4+5)"]
  w50 = FALSE ("Front Panel Window:Show Menu Bar")
  # "Modo 4 (1+3+4+5) sumador A,B,C"
  # "Modo 4 (2+3+4+5) sumador A,B,C"
  # "Modo 4 (1+2+3+4) sumador A,B,C"
  # "Modo 3 (3+4+5) sumador A,B,C"
  # "Modo 3 (2+3+4) sumador A,B,C"
  # "Modo 3 (1+2+3) sumador A,B,C"
  # "Modo 2 (3+4) sumador A,B,C"
  # "Modo 2 (2+3) sumador A,B,C"
  # "Modo 2 (1+3) sumador A,B,C"
  # "max y min pero cogidos de la tabla en funcion\ndel numero de sumadores, por ejemplo si\nVin Asic es 200mV los limites tendremos que\ncogerlos para 400 mv (2 sumadores) 600 mv\n(3 sumadores) y 800 mv (4 sumadores)\nindices:\n0 100mv\n1 200mv\n2 300mv\n3 400mv\n4 500mv\n5 600mv\n6 700mv\n7 800mv\n\nasi que 200mv es el index 1 por eso le sumamos 1\nlo que da 2 y lo multiplicamos por el numero\nde sumadores 2,3,4 lo que nos da 4, 6, 8, a este index\nle restamos 1 y los indices finales son 3, 5, 7."
  # "Como no se puede comprobar cuando se produce la comparacion entre ADD A,B,C y su correspondiente VTH (LL Y HL) por las velocidades de comparacion,\nse procede ha realizar un truco, para lo cual establecemos 10.000 pulsos de entrada de unos 3 ns, repetido cada 1us y con una tension de entrada entre 100mV y 1V,\nluego procedemos a poner un valor en DAC_TH0...5 que produca que el comparador un disparo en su salida, consideramos que la tension DAC_TH es correcta cuando\nde los 10000 pulsos de entrada 5000 disparan el comparador.\nPara poner la tension de entrada podriamos incremetar de 1 en 1 hasta obtener este valor.... MAL. realizamos un registro de aproximacion sucesivas (SAR), de forma\nque empezamos con DAC_TH 1000 0000 PN=10 si el comparador da mas de 5000 pulsos ponemos el DAC_TH 0100 0000 PN=10 si da menos de 5000 pusos ponesmos\nel DAC_TH 1100 0000 PN=10 y asi sucesivamente hasta encontra el valor mas proximo a esos 5000 pulsos. \nLuego obtenemos el valor del DAC_TH y la tension en los pines del ASIC PTHT NTHT.\nLa diferencia con el test RATE SCAN anterior es que esta vez no solo activamos una entrada sino que activamos varias en funcion de esta tabla:\nModo 2: 1+3 .... 2+3 .... 4+3\nModo 3: 1+2+3 .... 2+3+4 .... 3+4+5\nModo 4: 1+2+3+4 .... 0+3+4+5 .... 2+3+4+5\nComo podemos deducir solo se activaran los interruptores necesarios en funcion del modo y procederemos a realizar la medida en todos los sumadores."
  # "Control_byte\nNum bit        Función\n0                     \"Escribir\" ADC\n1                      \"INIT_R\" ASIC (reset)\n2                      \"start_tx\" ASIC para configuración ASIC\n3                      \"enable\" para el pulso\n4                      \"actualizar\" para el pulso\n5                      \"Escribir_ganancia\" para configuración ganancia\n6                      \"start\" para apertura ventana temportal scalers\n\nLVDSByte\n0                        Input1 (de Scaler 1)\n1                        Input2 (de Scaler 2)"
  # "usb_reg1: out std_logic_vector(7 downto 0);-- control_byte\t\t\tgeneral para todos los bits sueltos de control\n\t\t\t  usb_reg2: out std_logic_vector(7 downto 0);-- input_vector_byte2 \tByte 2 de palabra configuración del ASIC\n\t\t\t  usb_reg3: out std_logic_vector(7 downto 0);-- input_vector_byte1 \tByte 1 de palabra configuración del ASIC\n\t\t\t  usb_reg4: out std_logic_vector(7 downto 0);-- input_vector_byte0 \tByte 0 de palabra configuración del ASIC\n\t\t\t  usb_reg5: out std_logic_vector(7 downto 0);-- DATA_byte_alto, \t\tentrada al ADCdriver\n\t\t\t  usb_reg6: out std_logic_vector(7 downto 0);-- DATA_byte_bajo, \t\tentrada al ADCdriver\n\t\t\t  usb_reg7: out std_logic_vector(7 downto 0);-- ganancia_VGA\t\t\tde configuración de la ganancia del VGA\n\t\t\t  usb_reg8: out std_logic_vector(7 downto 0);-- PulseLong_byte_alto\tpatrón del pulso de la VGA\n\t\t\t  usb_reg9: out std_logic_vector(7 downto 0);-- PulseLong_byte_bajo\n\t\t\t  usb_reg10: out std_logic_vector(7 downto 0);--Period_byte_alto\t\tperíodo de repetición del pulso de la VGA\n\t\t\t  usb_reg11: out std_logic_vector(7 downto 0);--Perido_byte_bajo\n\t\t\t  usb_reg12: out std_logic_vector(7 downto 0);--ventana_byte2\t\t\tSCALERS: ventana\n\t\t\t  usb_reg13: out std_logic_vector(7 downto 0);--ventana_byte1\t\n\t\t\t  usb_reg14: out std_logic_vector(7 downto 0);--ventana_byte0\n\t\t\t  usb_reg15: in std_logic_vector(7 downto 0);-- output_vector_byte_alto\tByte 1 de palabra de lectura que sale del ASIC\n\t\t\t  usb_reg16: in std_logic_vector(7 downto 0);-- output_vector_byte_bajo\tByte 0 de palabra de lectura que sale del ASIC\n\t\t\t  usb_reg17: in std_logic_vector(7 downto 0);-- output0_byte_alto\t\tSCALERS: salidas\n\t\t\t  usb_reg18: in std_logic_vector(7 downto 0);-- output0_byte_bajo\n\t\t\t  usb_reg19: in std_logic_vector(7 downto 0);-- output1_byte_alto\n\t\t\t  usb_reg20: in std_logic_vector(7 downto 0);-- output1_alto_bajo \n\t\t\t  usb_reg21: in std_logic_vector(7 downto 0);-- output2_byte_alto \n\t\t\t  usb_reg22: in std_logic_vector(7 downto 0);-- output2_alto_bajo \n\t\t\t  usb_reg23: in std_logic_vector(7 downto 0);-- para el canal_0 del ADCdriver\n\t\t\t  usb_reg24: in std_logic_vector(7 downto 0);\n\t\t\t  usb_reg25: in std_logic_vector(7 downto 0);-- para el canal_1 del ADCdriver\n\t\t\t  usb_reg26: in std_logic_vector(7 downto 0);\n\t\t\t  usb_reg27: in std_logic_vector(7 downto 0);-- para el canal_2 del ADCdriver\n\t\t\t  usb_reg28: in std_logic_vector(7 downto 0);\n\t\t\t  usb_reg29: in std_logic_vector(7 downto 0);-- para el canal_3 del ADCdriver\n\t\t\t  usb_reg30: in std_logic_vector(7 downto 0);\n\t\t\t  usb_reg31: in std_logic_vector(7 downto 0);-- para el canal_4 del ADCdriver\n\t\t\t  usb_reg32: in std_logic_vector(7 downto 0);\n\t\t\t  usb_reg33: in std_logic_vector(7 downto 0);-- para el canal_5 del ADCdriver\n\t\t\t  usb_reg34: in std_logic_vector(7 downto 0);\n\t\t\t  usb_reg35: in std_logic_vector(7 downto 0);-- para el canal_6 del ADCdriver\n\t\t\t  usb_reg36: in std_logic_vector(7 downto 0);\n\t\t\t  usb_reg37: in std_logic_vector(7 downto 0);-- para el canal_7 del ADCdriver\n\t\t\t  usb_reg38: in std_logic_vector(7 downto 0);\n\t\t\t  usb_reg39: in std_logic_vector(7 downto 0);-- para el canal_8 del ADCdriver\n\t\t\t  usb_reg40: in std_logic_vector(7 downto 0);\n\t\t\t  usb_reg41: in std_logic_vector(7 downto 0);-- para el canal_9 del ADCdriver\n\t\t\t  usb_reg42: in std_logic_vector(7 downto 0);\n\t\t\t  usb_reg43: in std_logic_vector(7 downto 0);-- para el canal_10 del ADCdriver\n\t\t\t  usb_reg44: in std_logic_vector(7 downto 0)--;  \n\n     usb_reg55 => LVDSByte"
  # "x 100000, que es lo mismo que dividir entre 10^-5ms"
  # "ventana de observación de los scalers en ms"
  # "a 100MHz, que es la velocidad del reloj general de la placa,\ncomo el período es 10^-5ms, para temporizar 50ms (ventana \nque con la tasa de inyección de pulsos de 200KHz contabiliza \n10000 pulsos) el valor hexadecimal de la ventana sería:\n4C4B40"
  n1 = disable-structure shown="Enabled" {
    frame Disabled {
      # "TARJETA 13 TIENE UN POCO MÁS DE \nRUIDO QUE LA 07, PORQUE HAY UN\nPOCO MÁS DE VARIABILIDAD EN LOS \nOFFSET ANALÓGICOS, AUNQUE SALEN\nSIMILARES"
      # "offset sumadores ASIC 373 calculado en tarjeta 13"
      # "offset sumadores ASIC 373 calculado en tarjeta 07"
      n2 = Transpose 2D Array(2D array=dbl[][] [[0.008, -0.023, -0.007], [0.013, -0.019, -0.003], [0.013, -0.019, -0.003], [0.019, -0.013, 0.002], [0.012, -0.019, -0.004], [0.02, -0.011, 0.004], [0.012, -0.019, -0.003]]) -> ()  [unwired: 1 out]
    }
    frame Enabled {
    }
  }
  n3 = call "TEST.TEMPERATURA.vi"("error IN"="Error IN", "input cluster"="Config Test IN") -> ("error out"=w5:errorcluster, "Temperatura"=w11:dbl, "OUT cluster 2"=w12:T2)  [unwired: 7 in]
  n4 = control-ref of="Operacion"() -> (w15:refnum<vi>)
  n5 = control-ref of="Debug"() -> ()  [unwired: 1 out]
  n6 = Unbundle By Name(w12) -> ("Config Test"=w55:T5, "Execucion Test.Vasic Actual"=w10:i32)
  n7 = Unbundle By Name(w12) -> ("Config Test"=w31:T5, "Result"=w33:T7, "Execucion Test.Vasic Actual"=w30:i32)
  n8 = Unbundle By Name(w12) -> ("Config HW.VISA Key 81160A"=w3:refnum<visa-resource-name>, "Config HW.Espera acceso FT"=w35:u32, "Config HW.FT_Handle"=w6:u32)  [unwired: 1 out]
  n9 = Unbundle By Name(w12) -> ("CONFIG GEN"=w4:T13[])
  n10 = control-ref of="This VI"() -> (w47:refnum<vi>)
  n11 = Index Array(array=w55, index=w10) -> (element=w54:T6)
  n12 = property class="VI"(reference=w47, "Front Panel.ShowMenuBar"=w50, "TB.Visible"=w50, "Front Panel.TitleBarVis"=TRUE ("Front Panel Window:Title Bar Visible"), "Front Panel.Title"="TEST ASIC. Rate Scan Adders" ("Front Panel Window:Title")) -> ()  [unwired: 1 in, 2 out]
  n13 = Index Array(array=w33, index=w30) -> (element=w32:T8)
  n14 = Index Array(array=w31, index=w30) -> (element=w29:T6)
  n15 = Unbundle By Name(w54) -> ("IBIAS"=w36:bool, "VALUE IBIAS"=w37:u8, "Vin Rate Adders"=w2:i32[], "Limits Rate Scan adders"=w45:cluster{"High":dbl[], "Low":dbl[]})
  n16 = Multiply(x=u32 10 ("Ventana"), y=u32 100000 ("Ventana")) -> (x*y=w66:u32)
  n17 = call "WINDOWS.AUTO SIZE.vi"("Error In"=w5, "TAB.AutoAjuste"=w15, "This VI"=w47) -> ()  [unwired: 4 in, 1 out]
  n18 = call "Scalers_Escribir ventana.vi"("Espera acceso USB"=w35, "error in"=w5, "Ventana"=w66, "ftHandle_in"=w6) -> ("error out"=w67:errorcluster, "ftHandle_out"=w68:u32)  [unwired: 6 in]
  n19 = call "ASIC_reset inicial.vi"("Espera acceso USB"=w35, "error in"=w67, "ftHandle_in"=w68) -> ("error out"=w38:errorcluster, "ftHandle_out"=w65:u32)  [unwired: 7 in]
  n20 = for {
    tunnel: w2 -> [w74] mode=indexing
    tunnel: w4 -> [w76]
    tunnel: [w73] -> w8 mode=indexing
    tunnel: [w72] -> w26 mode=indexing
    n21 = Index Array(array=w76, index=w74) -> (element=w75:T13)
    n22 = Unbundle By Name(w75) -> ("Amplitude"=w73:dbl, "Vasic Theorical"=w72:dbl)
  }
  "Vasic theo" <- w26
  "Vin real gen" <- w8
  n23 = Unbundle By Name(w32) -> ("Test Offset Analog add.V ADDOUT add"=w27:dbl[][])
  n24 = call "ASIC_CONFIGURAR IABIAS.vi"("Espera acceso USB"=w35, "error in"=w38, "IBIAS VALUE"=w37, "IBIAS"=w36, "ftHandle_in"=w65) -> ("error out"=w34:errorcluster, "ftHandle_out"=w39:u32)  [unwired: 5 in]
  n25 = Unbundle By Name(w45) -> ("High"=w44:dbl[], "Low"=w43:dbl[])
  n26 = for {
    tunnel: w44 -> [w89]
    tunnel: w43 -> [w88]
    tunnel: w2 -> [w87] mode=indexing
    tunnel: [w78] -> w42 mode=indexing
    tunnel: [w77] -> w41 mode=indexing
    n27 = Multiply(x=w87, y=3) -> (x*y=w85:i32)
    n28 = Index Array(array=w89, index #1=w85) -> (element #1=w84:dbl, element #2=w83:dbl, element #3=w82:dbl)  [unwired: 2 in]
    n29 = Index Array(array=w88, index #1=w85) -> (element #1=w81:dbl, element #2=w80:dbl, element #3=w79:dbl)  [unwired: 2 in]
    n30 = Build Array(w81, w81, w81, w80, w80, w80, w79, w79, w79) -> (w77:dbl[])
    n31 = Build Array(w84, w84, w84, w83, w83, w83, w82, w82, w82) -> (w78:dbl[])
  }
  "HIGH" <- w42
  "LOW" <- w41
  n32 = for "Tensiones Asic" {
    N -> [w122]
    tunnel: w35 -> [w129]
    tunnel: w66 -> [w138]
    tunnel: [w135] -> w61 mode=indexing
    tunnel: [w134] -> w60 mode=indexing
    tunnel: [w127] -> w25 mode=indexing
    tunnel: [w126] -> w24 mode=indexing
    tunnel: w8 -> [w109] mode=indexing
    tunnel: [w124] -> w53 mode=indexing
    tunnel: [w123] -> w52 mode=indexing
    tunnel: w26 -> [w121] mode=indexing
    shift-right: [w119] -> _
    shift-left: 0.0 ("x/y") -> [w120]
    shift-right: [w117] -> _
    shift-left: 0 -> [w118]
    tunnel: [w116] -> _
    tunnel: w27 -> [w115]
    tunnel: w39 -> [w130]
    tunnel: [w136] -> w63
    tunnel: w34 -> [w128]
    tunnel: [w108] -> w64
    tunnel: refnum<visa-resource-name> "USB0::0x0699::0x0408::C016316::INSTR" ("VISA Tek MDO3104") -> [w113]
    tunnel: [w106] -> w9 mode=indexing
    tunnel: w4 -> [w92]
    tunnel: w3 -> [w94]
    tunnel: w2 -> [w91] mode=indexing
    i -> [w93]
    stop <- w98 stop-if-true
    n33 = flat-sequence {
      tunnel: w95 -> [_]
      frame #0 {
        n34 = local write "Indicador"("Measuring real tension.\nPlease Wait." ("Indicador")) -> ()
      }
    }
    n35 = Index Array(array=w92, index=w91) -> (element=w90:T13)
    n36 = call "ADC_inicialización Setup-Averaging.vi"("ftHandle_in 2"=w130, "Espera acceso USB"=w129, "Reset (T=reset)"=TRUE, "Registro Setup (0x6800)"=u16 26624, "Registro Averaging (0x3200)"=u16 8192 ("Registro Setup (0x6800)"), "error in 2"=w128) -> ("ftHandle_out"=w97:u32, "error out"=w96:errorcluster)  [unwired: 8 in]
    n37 = call "configure generador FULL.vi"("error in"=w96, "Config Pulse"=w90, "VISA Key 81160A"=w94) -> ("error out"=w95:errorcluster)  [unwired: 6 in, 2 out]
    n38 = To Unsigned Byte Integer(number=w93) -> (unsigned 8bit integer=w125:u8)
    n39 = call "MISCELANEA_WAIT.vi"("ms wait IN"=u32 1000, "Error IN"=w95) -> ("Error OUT"=w112:errorcluster)  [unwired: 16 in, 1 out]
    n40 = call "Configure osciloscopio FULL con generador_ADDERS.vi"("Visa MDO3104"=w113, "Amplitud"=w109, "error out"=w112, "Esperar a completar estadisticas"=FALSE, "Configurar Osciloscopio"=TRUE) -> ("VISA resource name out 2"=w110:refnum<visa-resource-name>, "Math (CH1-CH2)"=w107:dbl, "error out 2"=w114:errorcluster)  [unwired: 6 in, 2 out]
    n41 = for "Modos de entrada (9)" {
      N: 9 -> [w149]
      tunnel: w129 -> [w162]
      tunnel: w138 -> [w163]
      tunnel: [w157] -> w135 mode=indexing
      tunnel: [w156] -> w134 mode=indexing
      tunnel: [w155] -> w127 mode=indexing
      tunnel: [w154] -> w126 mode=indexing
      tunnel: w125 -> [w153]
      tunnel: w107 -> [w152]
      tunnel: [w151] -> w124 mode=indexing
      tunnel: [w150] -> w123 mode=indexing
      tunnel: w122 -> [w148]
      tunnel: w121 -> [w147]
      shift-right: [w145] -> w119
      shift-left: w120 -> [w146]
      tunnel: [w144] -> w100
      shift-right: [w142] -> w117
      shift-left: w118 -> [w143]
      tunnel: [w141] -> w116
      tunnel: w115 -> [w140]
      tunnel: w97 -> [w166]
      tunnel: [w159] -> w136
      tunnel: w114 -> [w165]
      tunnel: [w158] -> w101
      i -> [w164]
      stop <- w144 stop-if-true
      n42 = To Unsigned Byte Integer(number=w164) -> (unsigned 8bit integer=w160:u8)
      n43 = for "Sumadores (3)" {
        N: 3 -> [w181]
        tunnel: w160 -> [w176]
        tunnel: w163 -> [w192]
        tunnel: w162 -> [w189]
        tunnel: [w194] -> w157 mode=indexing
        tunnel: [w193] -> w156 mode=indexing
        tunnel: [w184] -> w155 mode=indexing
        tunnel: [w186] -> w154 mode=indexing
        tunnel: w153 -> [w179]
        tunnel: w152 -> [w177]
        tunnel: [w185] -> w151 mode=indexing
        tunnel: [w183] -> w150 mode=indexing
        tunnel: w149 -> [w182]
        tunnel: w148 -> [w180]
        tunnel: w147 -> [w175]
        shift-right: [w173] -> w145
        shift-left: w146 -> [w174]
        tunnel: [w172] -> w144
        shift-right: [w167] -> w142
        shift-left: w143 -> [w170]
        tunnel: [w169] -> w141
        tunnel: w140 -> [w168]
        tunnel: w166 -> [w190]
        tunnel: [w188] -> w159
        tunnel: w165 -> [w191]
        tunnel: [w187] -> w158
        i -> [w178]
        stop <- w172 stop-if-true
        n44 = for "Intentos" {
          N: 1 -> [_]
          tunnel: [w206] -> w194
          tunnel: [w205] -> w193
          tunnel: w192 -> [w239]
          tunnel: w190 -> [w237]
          tunnel: w189 -> [w233]
          tunnel: [w232] -> w188
          tunnel: [w200] -> w186
          tunnel: [w229] -> w185
          tunnel: [w201] -> w184
          tunnel: [w228] -> w183
          tunnel: w182 -> [w226]
          tunnel: w181 -> [w225]
          tunnel: w180 -> [w224]
          tunnel: w179 -> [w223]
          tunnel: w178 -> [w220]
          tunnel: w177 -> [w196]
          tunnel: w176 -> [w199]
          tunnel: w175 -> [w215]
          tunnel: w174 -> [w213]
          tunnel: [w211] -> w173
          tunnel: [w197] -> w172
          shift-right: [w208] -> w167
          shift-left: w170 -> [w208]
          tunnel: [w203] -> w169
          tunnel: w168 -> [_]
          tunnel: w191 -> [w238]
          tunnel: [w231] -> w187
          i -> [w210]
          stop <- w197 stop-if-true
          w244 = TRUE  # Reset (T=reset)
          # "True, Gustavo, 23/07/2024"
          n45 = Compound Arithmetic op=MULTIPLY(w225, w226, w224) -> (w222:i32)
          n46 = To Unsigned Byte Integer(number=w220) -> (unsigned 8bit integer=w198:u8)
          n47 = Divide(x=100.0 ("value"), y=w222) -> (x/y=w212:dbl)
          n48 = Index Array(array=string[] ["A", "B", "C"], index=w220) -> (element=w219:string)
          n49 = Index Array(array=string[] ["MODE 2 (2+4)", "MODE 2 (3+4)", "MODE 2 (4+5)", "MODE 3 (2+3+4)", "MODE 3 (3+4+5)", "MODE 3 (4+5+6)", "MODE 4 (2+3+4+5)", "MODE 4 (3+4+5+6)", "MODE 4 (1+4+5+6)"] ("Column Headers"), index=w199) -> (element=w217:string)
          n50 = call "ASIC_Selecor canal Sumador (func sumas).vi"("Espera acceso USB"=w233, "error in"=w238, "Sumador"=w198, "Modo"=w199, "ftHandle_in"=w237) -> ("error out"=w236:errorcluster, "ftHandle_out"=w230:u32)  [unwired: 3 in, 2 out]
          n51 = Add(x=w212, y=w213) -> (x+y=w211:dbl)
          n52 = Bundle(cluster=T1 {"Sumador"=0, "Modo"=0, "Tension"=0, "Tension Real"=0.0}, "Sumador"=w198, "Modo"=w199, "Tension"=w223, "Tension Real"=w196) -> (w229:T1)
          "Ref" <- w229
          n53 = call "Barra puntos.vi"("#N"=w210) -> ("String"=w209:string)  [unwired: 8 in]
          n54 = call "ADC_inicialización Setup-Averaging.vi"("ftHandle_in 2"=w230, "Espera acceso USB"=w233, "Reset (T=reset)"=w244, "Registro Setup (0x6800)"=u16 26624, "Registro Averaging (0x3200)"=u16 8192 ("Registro Setup (0x6800)"), "error in 2"=w236) -> ("ftHandle_out"=w241:u32, "error out"=w240:errorcluster)  [unwired: 8 in]
          n55 = call "Rate scan.vi"("T Ventana"=w239, "Espera acceso USB"=w233, "error in 2"=w240, "Valor buscado scalers (5000)"=u16 5000 ("Valor buscado scalers"), "Sumador"=w198, "ftHandle_in 2"=w241) -> ("error out 2"=w234:errorcluster, "DAC\nTH3,TH4,TH5"=w205:u16, "DAC\nTH0,TH1,TH2"=w206:u16, "ftHandle_out 2"=w235:u32, "Scaler 1"=w228:u16)  [unwired: 1 in]
          "DAC TH0,TH1,TH2" <- w206
          "DAC TH3,TH4,TH5" <- w205
          n56 = local write "B"(w211) -> ()
          n57 = Format Into String(format string="VTheo %,;%1.4fV (Vreal %,;%1.4fV)\nMode %s Adder %s\n%sTotal Errors: %d%s", w215, w196, w217, w219, w209, w208, w209) -> (resulting string=w216:string)  [unwired: 2 in, 1 out]
          n58 = local write "%"(w211) -> ()
          n59 = local write "Indicador"(w216) -> ()
          n60 = case shown="False" TRUE {
            tunnel: w235 -> [w255 w267]
            tunnel: w234 -> [w250 w266]
            tunnel: w233 -> [w254 w257]
            tunnel: [w248 w265] -> w232
            tunnel: [w249 w264] -> w231
            tunnel: [w247 w263] -> w201
            tunnel: [w246 w262] -> w200
            tunnel: w198 -> [w253 w261]
            tunnel: w206 -> [w252 w260]
            tunnel: w205 -> [w251 w259]
            tunnel: [w254 w257] -> w203
            tunnel: [FALSE ("WRITE OK") w256] -> w195
            frame False {
              n61 = call "ASIC_WRITE THX THX3 READ ADC.vi"("ftHandle_in"=w255, "Sumador"=w253, "THX"=w252, "THX+3"=w251, "error in"=w250, "Espera acceso USB 2"=w254) -> ("ftHandle_out"=w248:u32, "HLTHx"=w247:dbl, "LLTHx"=w246:dbl, "error out"=w249:errorcluster)  [unwired: 10 in]
            }
            frame True {
              n62 = call "ADC_READ VHLTHx VLLTHx.vi"("ftHandle_out 2"=w267, "Sumador"=w261, "referenciar"=TRUE, "ref DAC\nTH0,TH1,TH2"=w260, "ref DAC\nTH3,TH4,TH5"=w259, "error out 2"=w266, "Espera acceso FT"=w257) -> ("WRITE OK"=w256:bool, "ftHandle_out"=w265:u32, "HLTHx"=w263:dbl, "LLTHx"=w262:dbl, "error out"=w264:errorcluster)  [unwired: 8 in]
            }
          }
          "HLTHx" <- w201
          "LLTHx" <- w200
          "WRITE OK" <- w195
          n63 = global read "Global.Salir Ya.vi" "Cancel"() -> (w197:bool)
        }
      }
    }
    n64 = Unbundle By Name(w101) -> ("status"=w99:bool)
    n65 = Or(x=w99, y=w100) -> (x .or. y?=w98:bool)
    n66 = call "Configure osciloscopio FULL con generador.vi"("Visa MDO3104"=w110, "Amplitud"=w109, "error out"=w101, "Esperar a completar estadisticas"=FALSE, "Configurar Osciloscopio"=FALSE) -> ("Math (CH1-CH2)"=w106:dbl, "error out 2"=w108:errorcluster)  [unwired: 6 in, 3 out]
    "Amplitude" <- w109
  }
  "DAC TH0,TH1,TH2 2" <- w61
  "DAC TH3,TH4,TH5 2" <- w60
  "Volt HLTH" <- w25
  "Volt LLTH" <- w24
  "Error OUT" <- w64
  n67 = Unbundle By Name(w29) -> ()  [unwired: 1 out]
  n68 = disable-structure shown="Enabled" {
    disable-tunnel: w8 -> [w268 _]
    disable-tunnel: [w268 w269] -> w7
    disable-tunnel: w9 -> [_ w269]
    frame Disabled {
    }
    frame Enabled {
    }
  }
  n69 = call "cruce por cero adders.vi"("Vin Asic Real"=w7, "Volt LLTH"=w24, "Volt HLTH"=w25) -> ("Volt LLTH Corregido"=w22:dbl[][][], "Cruce por 0 Salida b LLTH"=w21:dbl[][], "Cruce por 0 Salida a HLTH"=w20:dbl[][], "Volt HLTH Corregido"=w23:dbl[][][])  [unwired: 5 in]
  "Salida A rectificada" <- w23
  "Cruze por 0 Salida A" <- w20
  "Cruze por 0 Salida B" <- w21
  "Salida B rectificada" <- w22
  n70 = Unbundle By Name(w12) -> ("Result"=w58:T7, "Execucion Test.Vasic Actual"=w57:i32)
  n71 = for {
    tunnel: w23 -> [w271] mode=indexing
    tunnel: w22 -> [w270] mode=indexing
    tunnel: [w275] -> w18 mode=indexing
    tunnel: [w274] -> w19 mode=indexing
    tunnel: w42 -> [w273] mode=indexing
    tunnel: w41 -> [w272] mode=indexing
    n72 = for {
      tunnel: w271 -> [w281] mode=indexing
      tunnel: w270 -> [w280] mode=indexing
      tunnel: [w279] -> w275 mode=indexing
      tunnel: [w278] -> w274 mode=indexing
      tunnel: w273 -> [w277] mode=indexing
      tunnel: w272 -> [w276] mode=indexing
      n73 = In Range and Coerce(upper limit=w277, x=w280, lower limit=w276) -> (In Range?=w279:bool[])  [unwired: 1 out]
      n74 = In Range and Coerce(upper limit=w277, x=w281, lower limit=w276) -> (In Range?=w278:bool[])  [unwired: 1 out]
      "Volt HLTH Corregido" <- w281
      "Volt LLTH Corregido" <- w280
      "h8ig" <- w277
      "low" <- w276
    }
  }
  "Comparation HLTH" <- w19
  "Comparation LLTH" <- w18
  n75 = Index Array(array=w58, index=w57) -> (element=w62:T8)
  n76 = And Array Elements(Boolean array=w19) -> (logical AND=w16:bool)
  "logical AND" <- w16
  n77 = And Array Elements(Boolean array=w18) -> (logical AND=w17:bool)
  "logical AND 2" <- w17
  n78 = And(x=w16, y=w17) -> (x .and. y?=w51:bool)
  "Rate scan adders all ok" <- w51
  n79 = Bundle By Name(cluster=w62, "Test Rate Scan adders.Scaler 0"=w52, "Test Rate Scan adders.DAC TH0,TH1,TH2"=w61, "Test Rate Scan adders.DAC TH3,TH4,TH5"=w60, "Test Rate Scan adders.Volt HLTH"=w25, "Test Rate Scan adders.Volt LLTH"=w24, "Test Rate Scan adders.Add HLTH OK"=w19, "Test Rate Scan adders.Add LLTH 2 OK"=w18, "Test Rate Scan adders.Rate Scan Adders OK"=w51, "Test Rate Scan adders.Ref"=w53, "Test Rate Scan adders.OFFSET HLTH"=w20, "Test Rate Scan adders.OFFSET LLTH"=w21, "Test Rate Scan adders.Real Voltage"=w7, "info temp.T Asic Rate Scan Adders"=w11) -> (w59:T8)
  n80 = Insert Into Array(array=w58, index=w57, new element=w59) -> (w56:T7)
  n81 = Bundle By Name(cluster=w12, "Result"=w56, "Config HW.FT_Handle"=w63) -> (w28:T2)
  "Config Test OUT" <- w28
  n82 = disable-structure shown="Enabled" {
    disable-tunnel: w28 -> [w282 _]
    frame Enabled {
      n83 = flat-sequence {
        tunnel: w282 -> [_]
        frame #0 {
          n84 = control-ref of="This VI"() -> (w283:refnum<vi>)
          n85 = invoke class="VI" method="FP.Close"(reference=w283) -> ()  [unwired: 2 in, 3 out]
        }
      }
    }
    frame Disabled {
    }
  }
